vi "Analysis Cmd.vi"() -> ()   [LabVIEW 2019]
uses:
  Function/VisionSet/System/iVision/Controls/Parameter.ctl
  64e560cb-b4a6-4208-a2be-8d6ad7cbc757.vi
  <vilib>/JDP Science/JSONtext/JSON text to Variant.vi
  <vilib>/vision/NI_Vision_Development_Module.lvlib
panel:
  in  "Result Arr":refnum<vi>
  in  "CmdIn":string
  in  "CmdIndex":i32
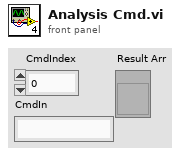
[diagram p1: front panel]
types:
  T1 = typedef "Parameter.ctl" = enum16{"Initialize", "Write", "Read", "WriteAll", "Save", "Load"}
  T2 = enum16{"Initial", "Write", "Read", "Save", "Load", "WrteAll"}
  T3 = cluster{"ROI":string, "Numbers":i32, "Data":string[][]}[]
  T4 = cluster{"ROI":string, "Numbers":i32, "Data":string[][]}
  T5 = typedef "ParameterData.ctl" = cluster{"Rotate Angle":dbl, "Rotate?":bool, "Calibration File Path":string, "Cal?":bool}
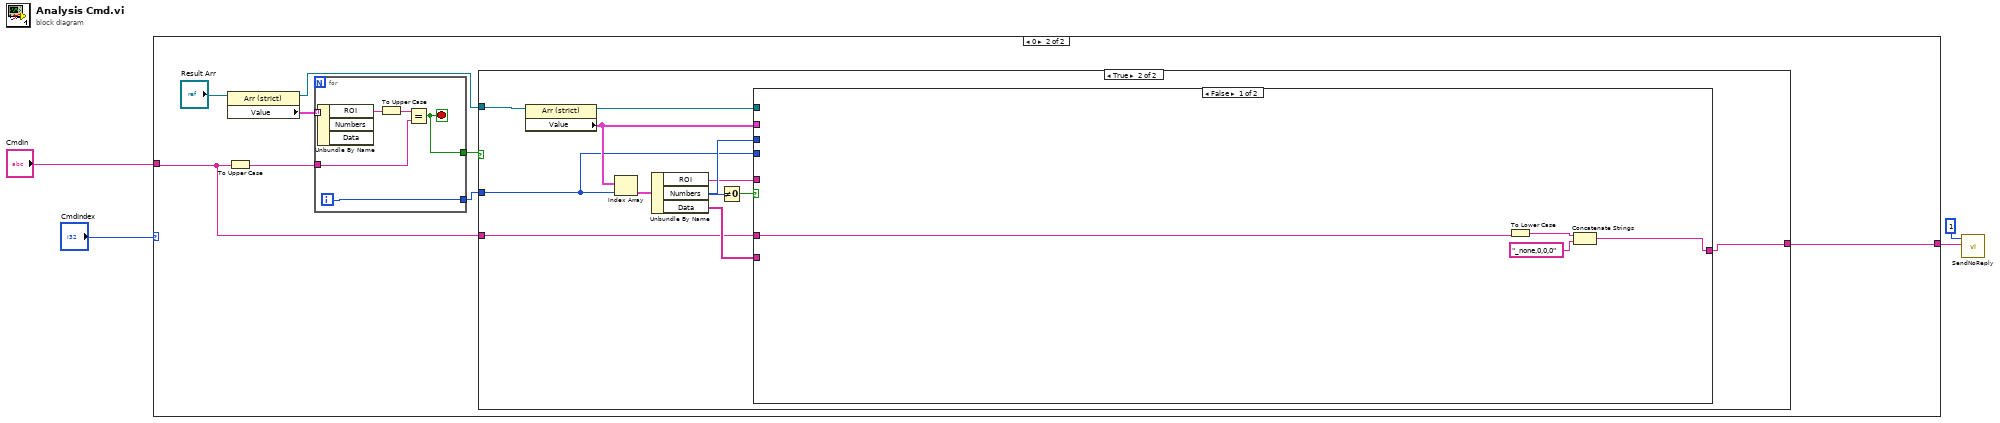
[diagram p0: block diagram]
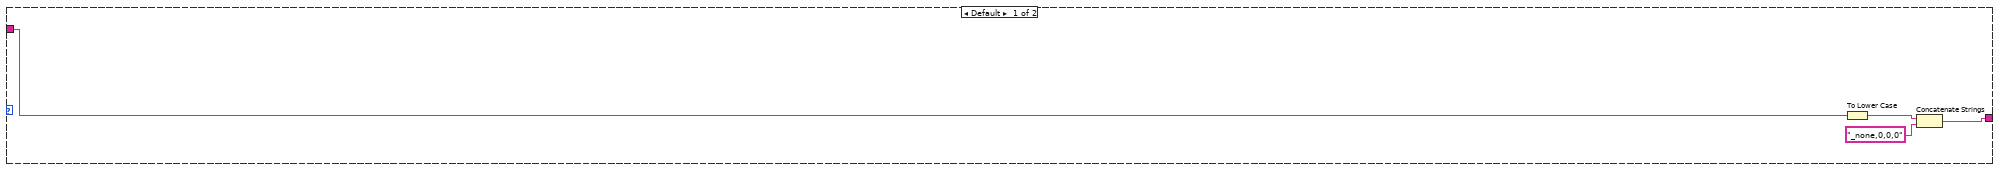
[diagram p2: hidden frame]
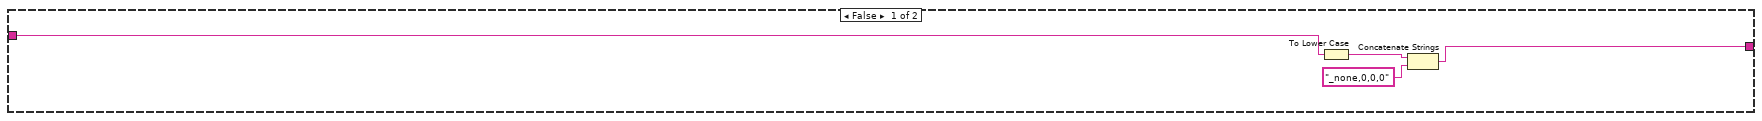
[diagram p3: hidden frame]
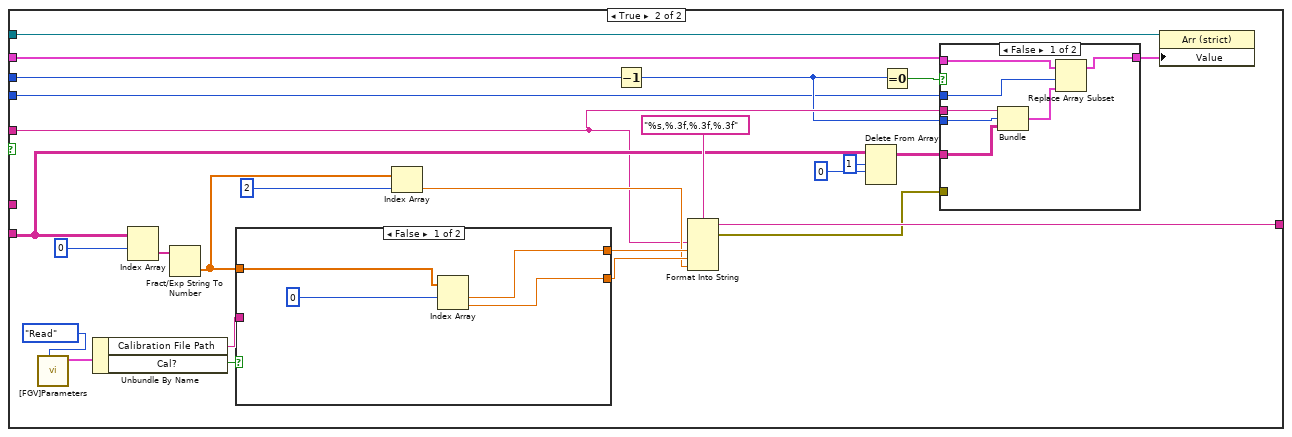
[diagram p4: hidden frame]
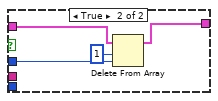
[diagram p5: hidden frame]
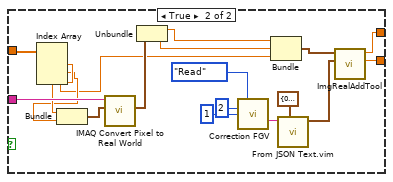
[diagram p6: hidden frame]
diagram:
  n1 = case shown="0" "CmdIndex" {
    tunnel: "CmdIn" -> [w5 w10]
    tunnel: [w6 w9] -> w2
    frame Default {
      n2 = To Lower Case(string=w5) -> (all lower case string=w8:string)
      n3 = Concatenate Strings(w8, "_none,0,0,0") -> (w6:string)
    }
    frame 0 {
      n4 = property class="Arr (strict)"(reference="Result Arr") -> (reference out=w12:refnum<vi>, "Value"=w15:T3)  [unwired: 1 in, 1 out]
      n5 = To Upper Case(1:w10) -> (0:w14:string)
      n6 = for {
        tunnel: w15 -> [w100] mode=indexing
        tunnel: w14 -> [w97]
        tunnel: [w96] -> w13
        tunnel: [w95] -> w11
        i -> [w95]
        stop <- w96 stop-if-true
        n7 = Unbundle By Name(w100) -> ("ROI"=w99:string)  [unwired: 2 out]
        n8 = To Upper Case(1:w99) -> (0:w98:string)
        n9 = Equal?(x=w98, y=w97) -> (x = y?=w96:bool)
      }
      n10 = case shown="True" w13 {
        tunnel: w12 -> [_ w24]
        tunnel: w11 -> [_ w22]
        tunnel: w10 -> [w18 w23]
        tunnel: [w17 w21] -> w9
        frame False {
          n11 = To Lower Case(string=w18) -> (all lower case string=w20:string)
          n12 = Concatenate Strings(w20, "_none,0,0,0") -> (w17:string)
        }
        frame True {
          n13 = property class="Arr (strict)"(reference=w24) -> (reference out=w29:refnum<vi>, "Value"=w31:T3)  [unwired: 1 in, 1 out]
          n14 = Index Array(array=w31, index=w22) -> (element=w25:T4)
          n15 = Unbundle By Name(w25) -> ("ROI"=w28:string, "Numbers"=w30:i32, "Data"=w27:string[][])
          n16 = Not Equal To 0?(x=w30) -> (x != 0?=w26:bool)
          n17 = case shown="False" w26 {
            tunnel: w27 -> [_ w48]
            tunnel: w28 -> [_ w40]
            tunnel: [w34 w50] -> w21
            tunnel: w29 -> [_ w45]
            tunnel: w30 -> [_ w49]
            tunnel: w31 -> [_ w43]
            tunnel: w23 -> [w33 _]
            tunnel: w22 -> [_ w36]
            frame False {
              n18 = To Lower Case(string=w33) -> (all lower case string=w32:string)
              n19 = Concatenate Strings(w32, "_none,0,0,0") -> (w34:string)
            }
            frame True {
              n20 = call "[FGV]Parameters.vi"("Parameter"=Parameter."Read") -> ("ParameterData Out"=w53:T5)  [unwired: 9 in, 1 out]
              n21 = Unbundle By Name(w53) -> ("Calibration File Path"=w37:string, "Cal?"=w51:bool)
              n22 = Index Array(array=w48, index (row)=0) -> (element=w60:string[])  [unwired: 1 in]
              n23 = Fract/Exp String To Number(string=w60) -> (number=w59:dbl[])  [unwired: 3 in, 1 out]
              n24 = case shown="False" w51 {
                tunnel: w59 -> [w75 w86]
                tunnel: [w74 w88] -> w56
                tunnel: [w73 w87] -> w55
                tunnel: w37 -> [_ w85]
                frame False {
                  n25 = Index Array(array=w75, index #1=0 ("index")) -> (element #1=w74:dbl, element #2=w73:dbl)  [unwired: 1 in]
                }
                frame True {
                  n26 = Index Array(array=w86) -> (element #1=w84:dbl, element #2=w83:dbl, element #3=w78:dbl)  [unwired: 3 in]
                  n27 = Bundle(w84, w83) -> (w82:cluster{dbl, dbl})  [unwired: 1 in]
                  n28 = call "IMAQ Convert Pixel to Real World"("Pixel Coordinates"=w82, "Calibrated Image"=w85) -> ("Real World Coordinates"=w81:cluster{"X":sgl, "Y":sgl})  [unwired: 4 in, 5 out]
                  n29 = Unbundle(w81) -> ("X"=w80:sgl, "Y"=w79:sgl)
                  n30 = call "Correction FGV.vi"("Action"=T2."Read", "X"=2, "Y"=1) -> ("DataOut"=w94:string)  [unwired: 10 in, 2 out]
                  n31 = Bundle("X"=w80, "Y"=w79, w78) -> (w77:cluster{"X":sgl, "Y":sgl, dbl})  [unwired: 1 in]
                  n32 = call "From JSON Text.vim"("Data Type and Default Value"=cluster{"X":dbl, "Y":dbl, "Angle":dbl} {"X"=0.0, "Y"=0.0, "Angle"=0.0} ("ToolData"), "JSON"=w94) -> ("Data out"=w89:cluster{"X":dbl, "Y":dbl, "Angle":dbl})  [unwired: 8 in, 1 out]
                  n33 = call "ImgRealAddTool.vi"("ToolData"=w89, "ImgRealData"=w77) -> ("YFinal"=w87:dbl, "XFinal"=w88:dbl)  [unwired: 8 in]
                }
              }
              n34 = Index Array(array=w59, index=2) -> (element=w54:dbl)
              n35 = Decrement(x=w49) -> (x-1=w39:i32)
              n36 = Format Into String(format string="%s,%.3f,%.3f,%.3f", w40, w56, w55, w54) -> (resulting string=w50:string, error out=w41:errorcluster)  [unwired: 2 in]
              n37 = Delete From Array(array=w48, length=1, index (row)=0) -> (array with subset deleted=w38:string[][])  [unwired: 1 in, 1 out]
              n38 = Equal To 0?(x=w39) -> (x = 0?=w44:bool)
              n39 = case shown="False" w44 {
                tunnel: w43 -> [w67 w71]
                tunnel: [w68 w70] -> w42
                tunnel: w41 -> [_ _]
                tunnel: w40 -> [w66 _]
                tunnel: w39 -> [w65 _]
                tunnel: w38 -> [w64 _]
                tunnel: w36 -> [w62 w69]
                frame False {
                  n40 = Bundle("ROI"=w66, w65, "Data"=w64) -> (w63:cluster{"ROI":string, i32, "Data":string[][]})  [unwired: 1 in]
                  n41 = Replace Array Subset(array=w67, new element=w63, index=w62) -> (w68:T3)
                }
                frame True {
                  n42 = Delete From Array(array=w71, length=1, index=w69) -> (array with subset deleted=w70:T3)  [unwired: 1 out]
                }
              }
              n43 = property class="Arr (strict)"(reference=w45, "Value"=w42) -> ()  [unwired: 1 in, 2 out]
            }
          }
        }
      }
    }
  }
  n44 = call "SendNoReply.vi"("DataIn"=w2, "index"=1) -> ()  [unwired: 9 in, 1 out]
